vi "REL_Move(PIC).vi"(3 "baud rate (9600)":u32=115200 caption="보 전송속도(9600)", 4 "X Position(REL)":dbl format="%#_8g", 5 "Y Position(REL)":dbl format="%#_8g", 6 "Port":refnum<visa-resource-name>="COM4" caption="VISA 리소스 이름") -> (0 "에러 출력":errorcluster, 2 "VISA 리소스 이름 출력":refnum<visa-resource-name>)   [LabVIEW 2010]
uses:
  <vilib>/Instr/_visa.llb/VISA Flush IO Buffer Mask.ctl
  <vilib>/Instr/_visa.llb/VISA Configure Serial Port (Instr).vi
panel:
  out "연결된 문자열":string
  out "Write data":u32
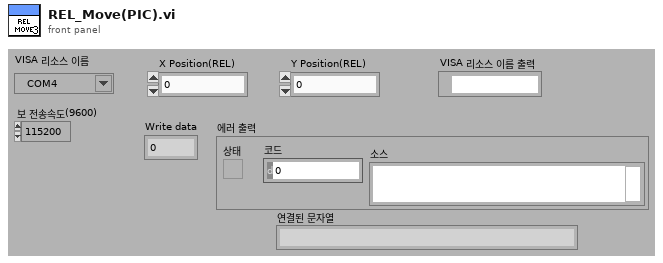
[diagram p1: front panel]
types:
  T1 = typedef "VISA Flush IO Buffer Mask.ctl" = u16
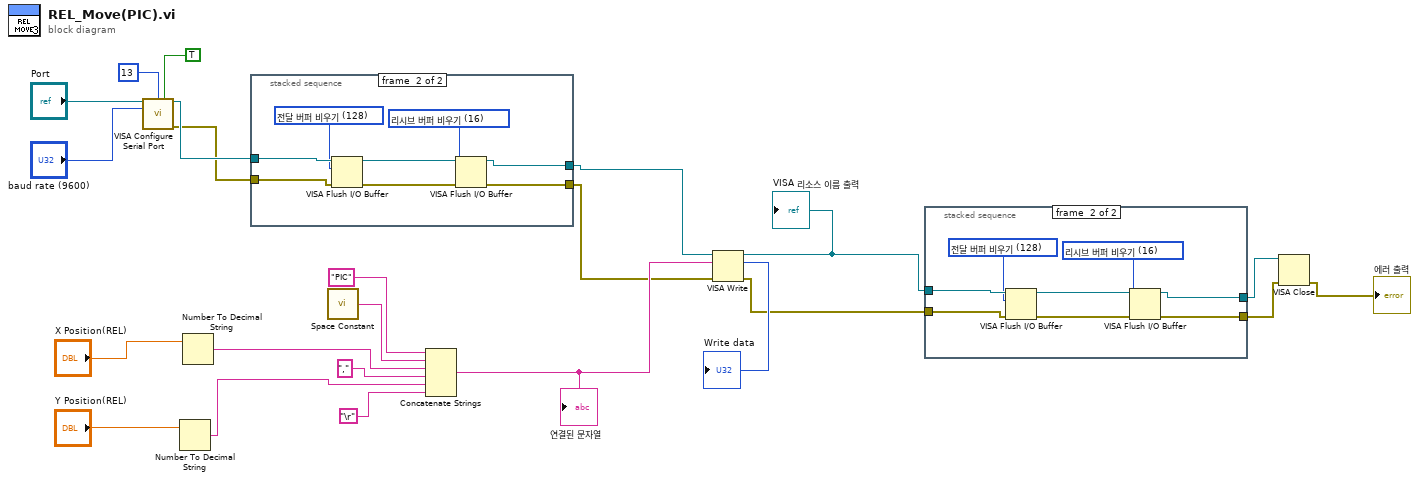
[diagram p0: block diagram]
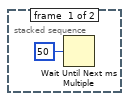
[diagram p2: hidden frame]
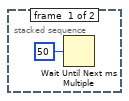
[diagram p3: hidden frame]
diagram:
  n1 = call-poly "VISA Configure Serial Port"("VISA resource name"="Port", "termination char\n(0xA = '\\n' = LF)"=i16 13 ("termination char\n(0xA = '\\n' = LF)"), "Enable Termination\nChar (T)"=TRUE ("Enable Termination\nChar (T)"), "baud rate (9600)"="baud rate (9600)") -> ("VISA resource name out"=w2:refnum<visa-resource-name>, "error out"=w1:errorcluster)  [unwired: 10 in]
  n2 = Number To Decimal String(number="Y Position(REL)") -> (decimal integer string=w15:string)  [unwired: 1 in]
  n3 = Number To Decimal String(number="X Position(REL)") -> (decimal integer string=w17:string)  [unwired: 1 in]
  n4 = stacked-sequence {
    tunnel: w2 -> [_ w32]
    tunnel: w1 -> [_ w31]
    tunnel: [_ w27] -> w4
    tunnel: [_ w26] -> w3
    frame #0 {
      n5 = Wait Until Next ms Multiple(millisecond multiple=u32 50 ("ms 배수")) -> ()  [unwired: 1 out]
    }
    frame #1 {
      w25 = T1 16 items=["리시브 버퍼 비우기"=16, "전달 버퍼 디바이스에 쓰기"=32, "리시브 버퍼 비우기(I/O 없음)"=64, "전달 버퍼 비우기"=128] ("Mask")
      w30 = T1 128 items=["리시브 버퍼 비우기"=16, "전달 버퍼 디바이스에 쓰기"=32, "리시브 버퍼 비우기(I/O 없음)"=64, "전달 버퍼 비우기"=128] ("Mask")
      n6 = VISA Flush I/O Buffer(VISA resource name=w32, mask (16)=w30, error in (no error)=w31) -> (VISA resource name out=w29:refnum<visa-resource-name>, error out=w28:errorcluster)
      n7 = VISA Flush I/O Buffer(VISA resource name=w29, mask (16)=w25, error in (no error)=w28) -> (VISA resource name out=w27:refnum<visa-resource-name>, error out=w26:errorcluster)
    }
  }
  n8 = call <vilib>:"Space Constant.vi"() -> ("String"=w18:string)
  n9 = Concatenate Strings("PIC" ("버퍼 쓰기"), w18, w17, "," ("문자열"), w15, "\r") -> (w21:string)
  "연결된 문자열" <- w21
  n10 = VISA Write(VISA resource name=w4, write buffer=w21, error in (no error)=w3) -> (VISA resource name out=w8:refnum<visa-resource-name>, return count=→"Write data":u32, error out=w7:errorcluster)
  "VISA 리소스 이름 출력" <- w8
  n11 = stacked-sequence {
    tunnel: w8 -> [_ w41]
    tunnel: w7 -> [_ w40]
    tunnel: [_ w36] -> w6
    tunnel: [_ w35] -> w5
    frame #0 {
      n12 = Wait Until Next ms Multiple(millisecond multiple=u32 50 ("ms 배수")) -> ()  [unwired: 1 out]
    }
    frame #1 {
      w34 = T1 16 items=["리시브 버퍼 비우기"=16, "전달 버퍼 디바이스에 쓰기"=32, "리시브 버퍼 비우기(I/O 없음)"=64, "전달 버퍼 비우기"=128] ("Mask")
      w39 = T1 128 items=["리시브 버퍼 비우기"=16, "전달 버퍼 디바이스에 쓰기"=32, "리시브 버퍼 비우기(I/O 없음)"=64, "전달 버퍼 비우기"=128] ("Mask")
      n13 = VISA Flush I/O Buffer(VISA resource name=w41, mask (16)=w39, error in (no error)=w40) -> (VISA resource name out=w38:refnum<visa-resource-name>, error out=w37:errorcluster)
      n14 = VISA Flush I/O Buffer(VISA resource name=w38, mask (16)=w34, error in (no error)=w37) -> (VISA resource name out=w36:refnum<visa-resource-name>, error out=w35:errorcluster)
    }
  }
  n15 = VISA Close(VISA resource name=w6, error in (no error)=w5) -> (error out=→"에러 출력":errorcluster)
